vi "Initialize RT.vi"(8 "error in (no error)":errorcluster) -> (0 "error out":errorcluster)   [LabVIEW 2015]
uses:
  <vilib>/nisyscfg/Find Hardware.vi
  <vilib>/nisyscfg/Close (System).vi
  <vilib>/nisyscfg/nisyscfg.lvlib
panel:
  out "size(s)":i32
  out "Resources out":refnum<k20>[](array[refnum])
  out "Numeric":i32
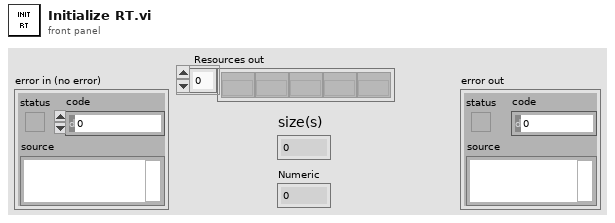
[diagram p1: front panel]
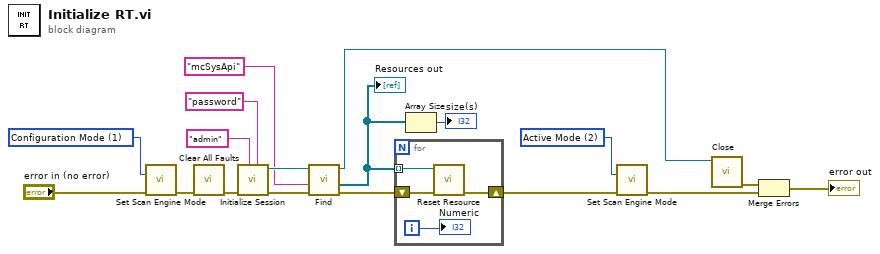
[diagram p0: block diagram]
diagram:
  w11 = 1 items=["Configuration Mode"=1, "Active Mode"=2] ("mode (Active Mode)")
  w15 = 2 items=["Configuration Mode"=1, "Active Mode"=2] ("mode (Active Mode)")
  n1 = call <vilib>:"Set Scan Engine Mode.vi"("mode (Active Mode)"=w11, "error in (no error)"="error in (no error)") -> ("error out"=w9:errorcluster)  [unwired: 13 in]
  n2 = call <vilib>:"Clear All Faults.vi"("error in (no error)"=w9) -> ("error out"=w17:errorcluster)  [unwired: 10 in]
  n3 = call <vilib>:"Initialize Session.vi"("Password"="password", "User Name"="admin", "error in (no error)"=w17) -> ("error out"=w18:errorcluster, "Session out"=w4:refnum<k21>)  [unwired: 7 in]
  n4 = call-poly <vilib>:"Find.vi"("error in (no error)"=w18, "Experts"="mcSysApi", "Session in"=w4) -> ("error out"=w14:errorcluster, "Resources out"=w8:refnum<k20>[], "Session out"=w5:refnum<k21>)  [unwired: 5 in, 1 out]
  "Resources out" <- w8
  n5 = for {
    tunnel: w8 -> [w21] mode=indexing
    shift-right: [w22] -> w16
    shift-left: w14 -> [w20]
    i -> [w19]
    n6 = call <vilib>:"Reset Resource.vi"("error in (no error)"=w20, "Resource in"=w21) -> ("error out"=w22:errorcluster)  [unwired: 6 in, 3 out]
    "Numeric" <- w19
  }
  n7 = Array Size(array=w8) -> (size(s)=→"size(s)":i32)
  n8 = call <vilib>:"Set Scan Engine Mode.vi"("mode (Active Mode)"=w15, "error in (no error)"=w16) -> ("error out"=w1:errorcluster)  [unwired: 13 in]
  n9 = call-poly <vilib>:"Close.vi"("Session in"=w5) -> ("error out"=w6:errorcluster)  [unwired: 10 in]
  n10 = Merge Errors(w6, w1) -> (→"error out":errorcluster)
